vi "clearpath_set_platform_name.vi"(0 "ClearpathComm":T1, 1 "New Name":string) -> ()   [LabVIEW 2012, in "clearpath_interface.lvlib"]
doc: "Formats a Set Platform Name command (0x2) given an input string. Uses the onboard Clearpath library to perform the actual message formatting."
uses:
  clearpath_interface.lvlib
  cwrap_crio.dll
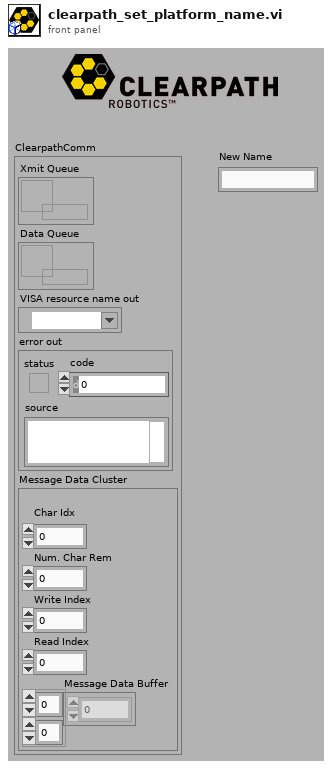
[diagram p1: front panel]
types:
  T1 = cluster{"Xmit Queue":refnum<queue>, "Data Queue":refnum<queue>, "VISA resource name out":refnum<visa-resource-name>, "error out":errorcluster, "Message Data Cluster":cluster{"\nChar Idx":u8, "Num. Char Rem":u8, "Write Index":u8, "Read Index":u8, "Message Data Buffer":u8[][]}}
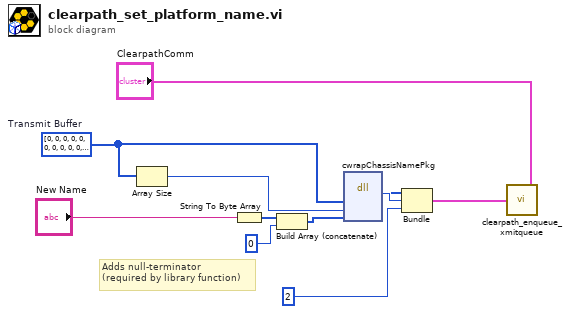
[diagram p0: block diagram]
diagram:
  w8 = u8[] [0, 0, 0, 0, 0, 0, 0, 0, 0, 0, 0, 0, 0, 0, 0, 0, 0, 0, 0, 0, 0, 0, 0, 0, 0, 0, 0, 0, 0, 0, 1, 0, 0, 0, 5]  # Transmit Buffer
  # "Adds null-terminator\n(required by library function)"
  n1 = Array Size(array=w8) -> (size(s)=w9:i32)
  n2 = String To Byte Array(string="New Name") -> (unsigned byte array=w6:u8[])
  n3 = Build Array (concatenate)(w6, u8 0) -> (w5:u8[])
  n4 = dll-call lib="C:/Users/tebbeam/Documents/GitHub/IGVC-2013/Code/Project 1.0/Motors/Husky/cwrap_cRIO.*" fn="cwrapChassisNamePkg"("buf"=w8, "buf_size"=w9, "name"=w5) -> ("return type"=w11:i32, "buf"=w10:u8[])  [unwired: 5 in, 2 out]
  n5 = Bundle("buf"=w10, "return type"=w11, 2) -> (w1:cluster{"buf":u8[], "return type":i32, i32})  [unwired: 1 in]
  n6 = call "clearpath_enqueue_xmitqueue.vi"("ClearpathComm"="ClearpathComm", "Cluster"=w1) -> ()
